vi "RunUpdater.vi"(8 "关闭前面板":bool, 9 "VI输入":refnum<vi>, 11 "run minimized? (F)":bool) -> ()   [LabVIEW 2015]
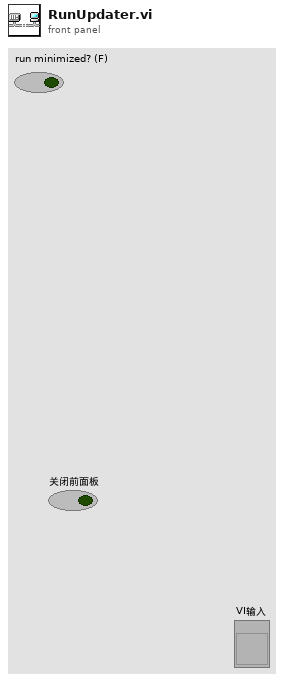
[diagram p1: front panel]
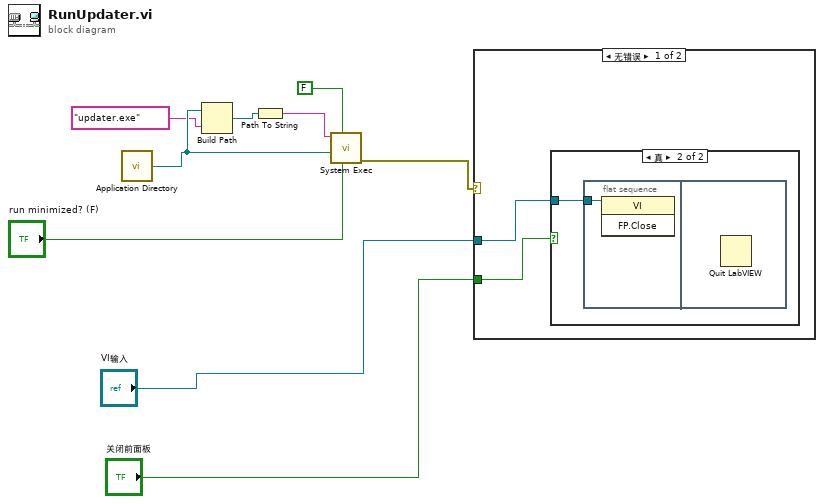
[diagram p0: block diagram]
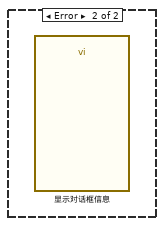
[diagram p3: hidden frame]
diagram:
  n1 = call <vilib>:"Application Directory.vi"() -> ("Application Directory"=w4:path)
  n2 = Build Path(base path=w4, name or relative path="updater.exe") -> (appended path=w5:path)
  n3 = Path To String(path=w5) -> (string=w6:string)
  n4 = call <vilib>:"System Exec.vi"("run minimized? (F)"="run minimized? (F)", "wait until completion? (T)"=FALSE, "working directory"=w4, "command line"=w6) -> ("error out"=w8:errorcluster)  [unwired: 4 in, 3 out]
  n5 = case shown="无错误" w8 {
    tunnel: "VI输入" -> [w11 _]
    tunnel: "关闭前面板" -> [w10 _]
    frame No Error {
      n6 = case shown="真" w10 {
        tunnel: w11 -> [_ w12]
        frame False {
        }
        frame True {
          n7 = flat-sequence {
            tunnel: w12 -> [w13]
            frame #0 {
              n8 = invoke class="VI" method="FP.Close"(reference=w13) -> ()  [unwired: 2 in, 3 out]
            }
            frame #1 {
              n9 = Quit LabVIEW() -> ()  [unwired: 1 in]
            }
          }
        }
      }
    }
    frame Error {
      n10 = call "显示对话框信息"() -> ()  [unwired: 10 in, 2 out]
    }
  }
